vi "Compact and Repair DB.vi"(4 "password (\"\")":string, 6 "username (\"\")":string, 8 "error in (no error)":errorcluster, 10 "Workgroup DB (none)":path, 11 "Database Path (empty)":path) -> (0 "error out":errorcluster)   [LabVIEW 2011]
uses:
  OpenG/file/file.llb/Strip Path Extension - String__ogtk.vi
  OpenG/file/file.llb/Valid Path - Traditional__ogtk.vi
panel:
  in  "JRO.IJetEngine":refnum<k7>
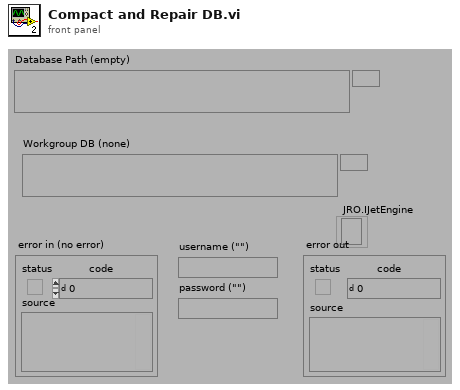
[diagram p1: front panel]
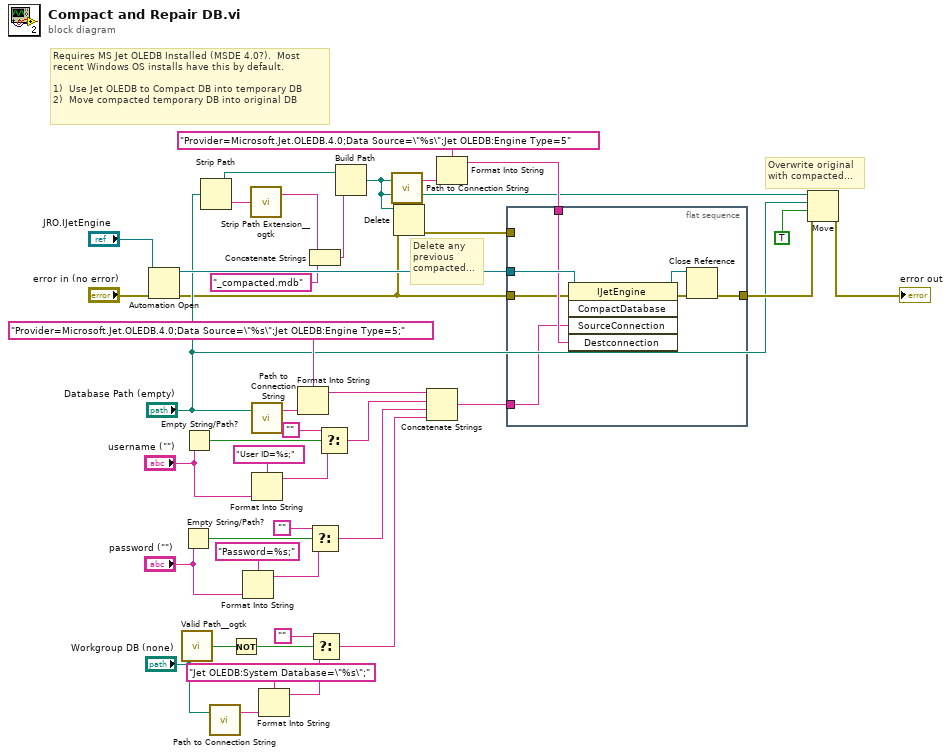
[diagram p0: block diagram]
diagram:
  # "Delete any\nprevious\ncompacted..."
  # "Overwrite original\nwith compacted..."
  # "Requires MS Jet OLEDB Installed (MSDE 4.0?).  Most\nrecent Windows OS installs have this by default.\n\n1)  Use Jet OLEDB to Compact DB into temporary DB\n2)  Move compacted temporary DB into original DB"
  n1 = Automation Open(error in (no error)="error in (no error)", Automation Refnum="JRO.IJetEngine") -> (Automation Refnum=w41:refnum<k7>, error out=w3:errorcluster)  [unwired: 2 out]
  n2 = call-poly "Valid Path__ogtk.vi"("path"="Workgroup DB (none)") -> ("valid"=w15:bool)
  n3 = Empty String/Path?(string/path="password (\"\")") -> (empty?=w28:bool)
  n4 = Empty String/Path?(string/path="username (\"\")") -> (empty?=w21:bool)
  n5 = Strip Path(path="Database Path (empty)") -> (stripped path=w6:path, name=w9:string)
  n6 = call "Path to Connection String.vi"("Path"="Workgroup DB (none)") -> ("Connection String"=w31:string)  [unwired: 2 out]
  n7 = Not(x=w15) -> (.not. x?=w11:bool)
  n8 = Format Into String(format string="Password=%s;" ("ConnectString"), "password (\"\")") -> (resulting string=w25:string)  [unwired: 2 in, 1 out]
  n9 = call-poly "Strip Path Extension__ogtk.vi"("path"=w9) -> ("root"=w8:string)  [unwired: 1 out]
  n10 = call "Path to Connection String.vi"("Path"="Database Path (empty)") -> ("Connection String"=w39:string)  [unwired: 2 out]
  n11 = Format Into String(format string="User ID=%s;" ("ConnectString"), "username (\"\")") -> (resulting string=w23:string)  [unwired: 2 in, 1 out]
  n12 = Format Into String(format string="Jet OLEDB:System Database=\"%s\";" ("ConnectString"), w31) -> (resulting string=w14:string)  [unwired: 2 in, 1 out]
  n13 = Format Into String(format string="Provider=Microsoft.Jet.OLEDB.4.0;Data Source=\"%s\";Jet OLEDB:Engine Type=5;" ("ConnectString"), w39) -> (resulting string=w24:string)  [unwired: 2 in, 1 out]
  n14 = Concatenate Strings(w8, "_compacted.mdb" ("Temporary File Extension (tmp)")) -> (w5:string)
  n15 = Select(t="", s=w28, f=w25) -> (s? t:f=w17:string)
  n16 = Select(t="", s=w11, f=w14) -> (s? t:f=w13:string)
  n17 = Select(t="", s=w21, f=w23) -> (s? t:f=w18:string)
  n18 = Build Path(base path=w6, name or relative path=w5) -> (appended path=w1:path)
  n19 = call "Path to Connection String.vi"("Path"=w1) -> ("Connection String"=w37:string)  [unwired: 2 out]
  n20 = Delete(path (use dialog)=w1, error in=w3) -> (error out=w2:errorcluster)  [unwired: 3 in, 2 out]
  n21 = Concatenate Strings(w24, w18, w17, w13) -> (w12:string)
  n22 = Format Into String(format string="Provider=Microsoft.Jet.OLEDB.4.0;Data Source=\"%s\";Jet OLEDB:Engine Type=5" ("ConnectString"), w37) -> (resulting string=w36:string)  [unwired: 2 in, 1 out]
  n23 = flat-sequence {
    tunnel: w41 -> [w49]
    tunnel: w36 -> [w46]
    tunnel: [w45] -> w35
    tunnel: w12 -> [w44]
    tunnel: w3 -> [w43]
    tunnel: w2 -> [_]
    frame #0 {
      n24 = invoke class="IJetEngine" method="CompactDatabase"(reference=w49, error in=w43, "SourceConnection"=w44, "Destconnection"=w46) -> (reference out=w47:refnum<k7>, error out=w48:errorcluster)  [unwired: 1 in, 3 out]
      n25 = Close Reference(reference=w47, error in (no error)=w48) -> (error out=w45:errorcluster)
    }
  }
  n26 = Move(source path=w1, error in=w35, 9:TRUE, 10:"Database Path (empty)") -> (error out=→"error out":errorcluster)  [unwired: 3 out]
